vi "star pattern.vi"() -> ()   [LabVIEW 2025]
panel:
  out "Pyramid pattern":string
  out "star":string
  out "concatenated string":string
  out "Middle star pattern":string
  out "string pattern":string
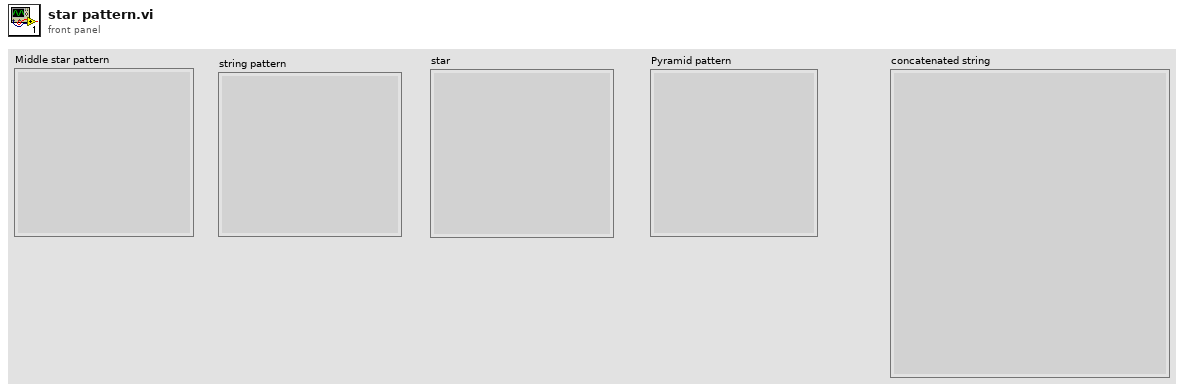
[diagram p1: front panel]
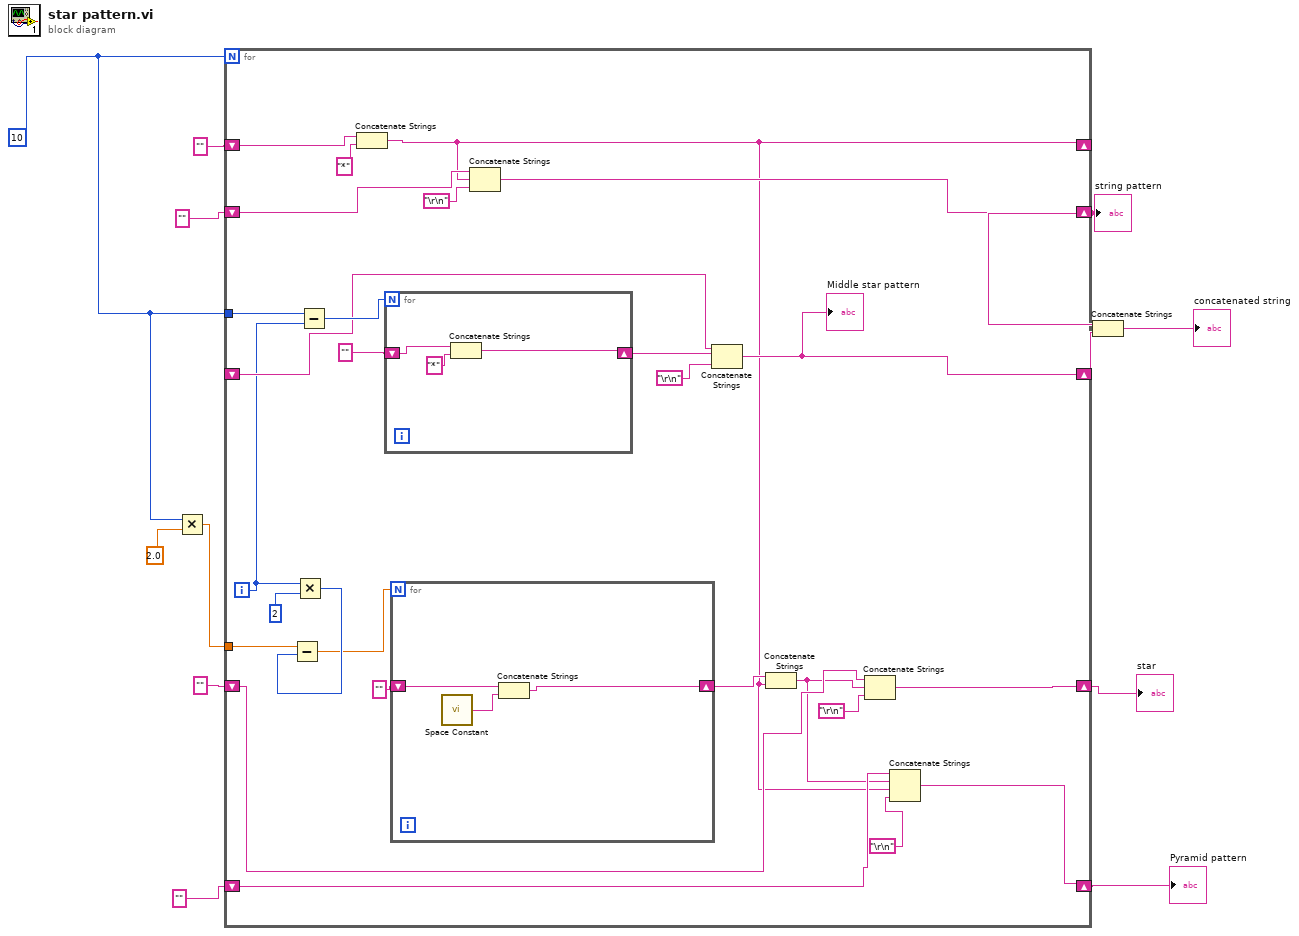
[diagram p0: block diagram]
diagram:
  w6 = 10
  n1 = Multiply(x=w6, y=2.0) -> (x*y=w5:dbl)
  n2 = for {
    N: w6 -> [_]
    shift-right: [w14] -> _
    shift-left: "" -> [w38]
    shift-right: [w35] -> w9
    shift-left: "" -> [w36]
    tunnel: w6 -> [w34]
    shift-right: [w28] -> w10
    shift-left: _ -> [w29]
    tunnel: w5 -> [w25]
    shift-right: [w19] -> w3
    shift-left: "" -> [w20]
    shift-right: [w16] -> w1
    shift-left: "" -> [w17]
    i -> [w27]
    n3 = Multiply(x=w27, y=2) -> (x*y=w26:i32)
    n4 = Subtract(x=w25, y=w26) -> (x-y=w24:dbl)
    n5 = Subtract(x=w34, y=w27) -> (x-y=w33:i32)
    n6 = Concatenate Strings(w38, "*" ("string")) -> (w14:string)
    n7 = for {
      N: w33 -> [_]
      shift-right: [w43] -> w31
      shift-left: "" -> [w44]
      n8 = Concatenate Strings(w44, "*" ("string")) -> (w43:string)
    }
    n9 = for {
      N: w24 -> [_]
      shift-right: [w40] -> w22
      shift-left: "" -> [w41]
      n10 = call <vilib>:"Space Constant.vi"() -> ("String"=w42:string)
      n11 = Concatenate Strings(w41, w42) -> (w40:string)
    }
    n12 = Concatenate Strings(w36, w14, "\r\n") -> (w35:string)
    n13 = Concatenate Strings(w29, w31, "\r\n") -> (w28:string)
    "Middle star pattern" <- w28
    n14 = Concatenate Strings(w22, w14) -> (w15:string)
    n15 = Concatenate Strings(w20, w15, "\r\n") -> (w19:string)
    n16 = Concatenate Strings(w17, w15, w14, "\r\n") -> (w16:string)
  }
  "string pattern" <- w9
  "star" <- w3
  "Pyramid pattern" <- w1
  n17 = Concatenate Strings(w9, w10) -> (→"concatenated string":string)
